vi "RPT Comaristion.vi"(10 "True":bool) -> (1 "Fail":bool)   [LabVIEW 2015]
uses:
  Galobal variable_TI.vi
  Project Setup/Globle Variable/GR_Servo.vi
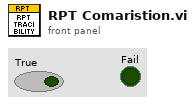
[diagram p1: front panel]
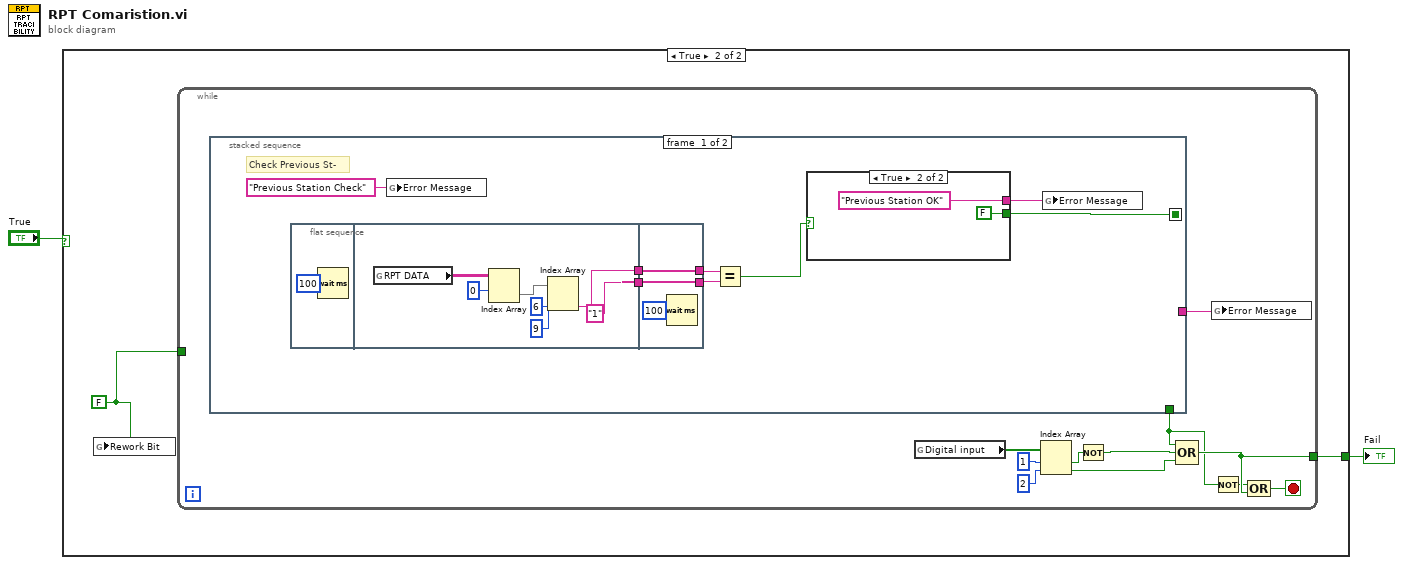
[diagram p0: block diagram]
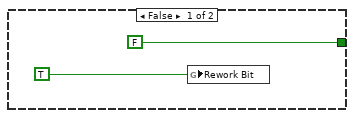
[diagram p2: hidden frame]
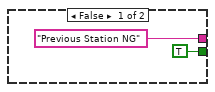
[diagram p3: hidden frame]
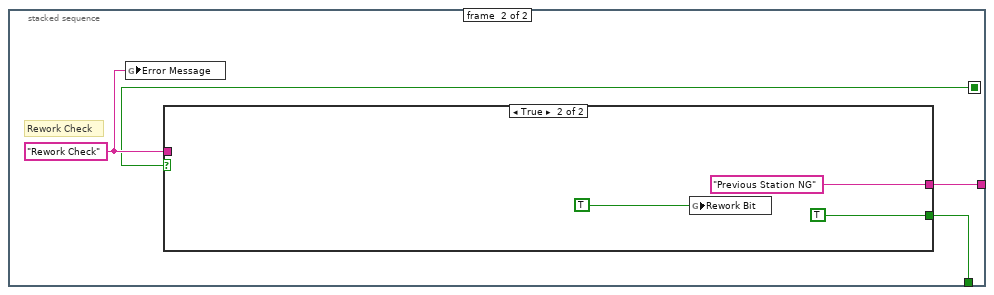
[diagram p4: hidden frame]
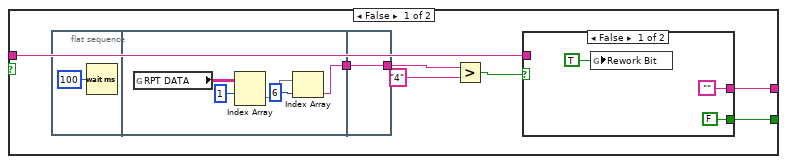
[diagram p5: hidden frame]
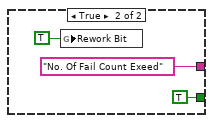
[diagram p6: hidden frame]
diagram:
  n1 = case shown="True" "True" {
    tunnel: [FALSE w6] -> w1
    frame False {
      n2 = global write "Galobal variable_TI.vi" "Rework Bit"(TRUE ("Rework bit")) -> ()
    }
    frame True {
      w5 = FALSE ("Rework bit")
      n3 = global write "Galobal variable_TI.vi" "Rework Bit"(w5) -> ()
      n4 = while {
        tunnel: [w10] -> w6
        tunnel: w5 -> [_]
        stop <- w11 stop-if-true
        n5 = stacked-sequence {
          seq-local: [w21 _] -> [_ w43]
          tunnel: [_ w42] -> w9
          tunnel: [_ w41] -> w8
          frame #0 {
            # "Check Previous St-"
            n6 = flat-sequence {
              tunnel: ["1" ("y")] -> w19
              tunnel: [w27] -> w18
              tunnel: [w35] -> w20
              tunnel: [w36] -> w25
              tunnel: w19 -> [w36]
              tunnel: w18 -> [w35]
              frame #0 {
                n7 = Wait (ms)(milliseconds to wait=u32 100) -> ()  [unwired: 1 out]
              }
              frame #1 {
                n8 = global read "GR_Servo.vi" "RPT DATA"() -> (w29:string[][])
                n9 = Index Array(array=w29, index (row)=0) -> (element=w31:string[])  [unwired: 1 in]
                n10 = Index Array(array=w31, index #1=6 ("index"), index #2=9 ("index")) -> (element #2=w27:string)  [unwired: 1 out]
              }
              frame #2 {
                n11 = Wait (ms)(milliseconds to wait=u32 100) -> ()  [unwired: 1 out]
              }
            }
            n12 = global write "GR_Servo.vi" "Error Message"("Previous Station Check") -> ()
            n13 = Equal?(x=w20, y=w25) -> (x = y?=w22:bool)
            n14 = case shown="True" w22 {
              tunnel: ["Previous Station NG" "Previous Station OK"] -> w23
              tunnel: [TRUE FALSE] -> w21
              frame False {
              }
              frame True {
              }
            }
            n15 = global write "GR_Servo.vi" "Error Message"(w23) -> ()
          }
          frame #1 {
            w44 = "Rework Check"
            # "Rework Check"
            n16 = global write "GR_Servo.vi" "Error Message"(w44) -> ()
            n17 = case shown="True" w43 {
              tunnel: w44 -> [w48 _]
              tunnel: [w47 "Previous Station NG"] -> w42
              tunnel: [w46 TRUE] -> w41
              frame False {
                n18 = flat-sequence {
                  tunnel: [w54] -> w45
                  tunnel: [w58] -> w50
                  tunnel: w45 -> [w58]
                  frame #0 {
                    n19 = Wait (ms)(milliseconds to wait=u32 100) -> ()  [unwired: 1 out]
                  }
                  frame #1 {
                    n20 = global read "GR_Servo.vi" "RPT DATA"() -> (w55:string[][])
                    n21 = Index Array(array=w55, index (row)=1) -> (element=w57:string[])  [unwired: 1 in]
                    n22 = Index Array(array=w57, index=6) -> (element=w54:string)
                  }
                  frame #2 {
                  }
                }
                n23 = Greater?(x=w50, y="4") -> (0:w49:bool)
                n24 = case shown="False" w49 {
                  tunnel: ["" "No. Of Fail Count Exeed"] -> w47
                  tunnel: w48 -> [_ _]
                  tunnel: [FALSE TRUE] -> w46
                  frame False {
                    n25 = global write "Galobal variable_TI.vi" "Rework Bit"(TRUE) -> ()
                  }
                  frame True {
                    n26 = global write "Galobal variable_TI.vi" "Rework Bit"(TRUE) -> ()
                  }
                }
              }
              frame True {
                n27 = global write "Galobal variable_TI.vi" "Rework Bit"(TRUE ("Rework bit")) -> ()
              }
            }
          }
        }
        n28 = global read "Galobal variable_TI.vi" "Digital input"() -> (w17:bool[])
        n29 = Index Array(array=w17, index #1=1 ("index"), index #2=2 ("index")) -> (element #1=w14:bool, element #2=w12:bool)
        n30 = Not(x=w14) -> (.not. x?=w13:bool)
        n31 = Compound Arithmetic op=OR(w8, w13, w12) -> (w10:bool)
        n32 = global write "GR_Servo.vi" "Error Message"(w9) -> ()
        n33 = Not(x=w8) -> (.not. x?=w7:bool)
        n34 = Compound Arithmetic op=OR(w7, w10) -> (w11:bool)
      }
    }
  }
  "Fail" <- w1
